vi "Write Instance Name.vi"(8 "error in (no error)":errorcluster, 10 "Instance Name":string, 11 "System Actor in":refnum<class "System Actor.lvclass">) -> (0 "error out":errorcluster, 3 "System Actor out":refnum<class "System Actor.lvclass">)   [LabVIEW 2014, in "Robot Actor Framework.lvlib" / "System Actor.lvlib" / "System Actor.lvclass"]
uses:
  System Actor.lvclass
  System Actor.lvclass/System Actor.ctl
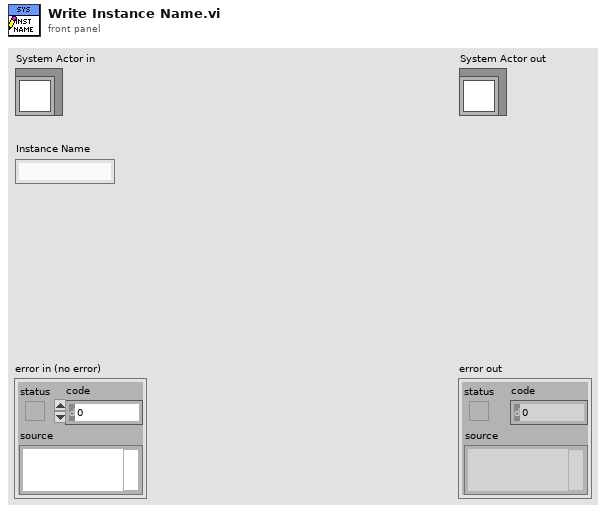
[diagram p1: front panel]
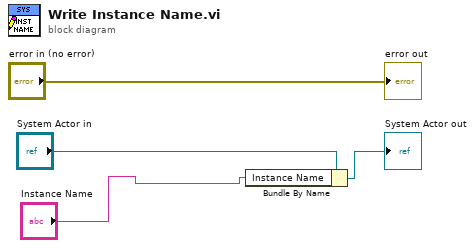
[diagram p0: block diagram]
diagram:
  n1 = Bundle By Name(cluster="System Actor in", "Instance Name"="Instance Name") -> (→"System Actor out":refnum<class "System Actor.lvclass">)
  "error out" <- "error in (no error)"
